vi "AppConfigFilePath.vi"() -> (3 "App Settings Path":path)   [LabVIEW 2015, in "AppConfig.lvlib"]
uses:
  AppConfig.lvlib
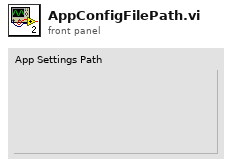
[diagram p1: front panel]
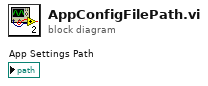
[diagram p0: block diagram]
diagram:
